vi "_Write.vi"(8 "error in (no error)":errorcluster, 10 "Data":string, 11 "TCP Stream in":refnum<class "TCP Stream.lvclass">) -> (0 "error out":errorcluster, 3 "TCP Stream out":refnum<class "TCP Stream.lvclass">)   [LabVIEW 2020, in "Stream-TCP.lvlib" / "TCP Stream.lvclass"]
uses:
  TCP Stream.lvclass
  TCP Stream.lvclass/TCP Stream.ctl
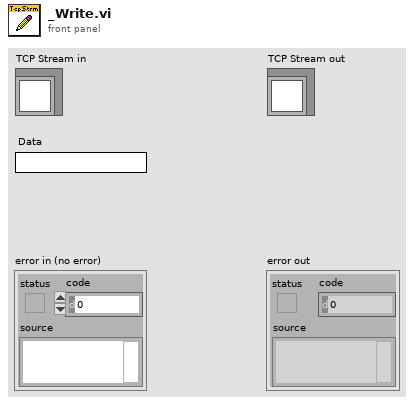
[diagram p1: front panel]
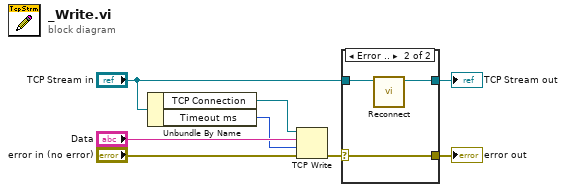
[diagram p0: block diagram]
diagram:
  n1 = Unbundle By Name("TCP Stream in") -> ("TCP Connection"=w8:refnum<k5>, "Timeout ms"=w4:i32)
  n2 = TCP Write(connection ID=w8, data in="Data", error in (no error)="error in (no error)", 9:w4) -> (error out=w6:errorcluster)  [unwired: 2 out]
  n3 = case shown="Error .." w6 {
    selector: w6 -> [w9 w12]
    tunnel: "TCP Stream in" -> [w10 w13]
    tunnel: [w9 w12] -> w2
    tunnel: [w10 w11] -> w5
    frame No Error {
    }
    frame Error {
      n4 = call "Reconnect.vi"("TCP Stream in"=w13) -> ("TCP Stream out"=w11:refnum<class "TCP Stream.lvclass">)  [unwired: 9 in, 1 out]
    }
  }
  "error out" <- w2
  "TCP Stream out" <- w5
